vi "Configure Reference Wavelength.vi"(6 "Reference Wavelength (0 nm)":dbl, 7 "Channel (1: Channel 1)":i32(ring)=1 items=["All"=0, "Channel 1"=1, "Channel 1.1"=11, "Channel 1.2"=12, "Channel 1.3"=13, "Channel 1.4"=14, "Channel 2"=2, "Channel 2.1"=21, "Channel 2.2"=22, "Channel 2.3"=23, "Channel 2.4"=24, "Channel 3"=3, "Channel 3.1"=31, "Channel 3.2"=32, "Channel 3.3"=33, "Channel 3.4"=34, "Channel 4"=4, "Channel 4.1"=41, "Channel 4.2"=42, "Channel 4.3"=43, "Channel 4.4"=44], 8 "error in (no error)":errorcluster, 9 "Reference Action (0:Enable)":u16(ring) items=["Enable", "Disable", "Clear"], 10 "Sensor Number (1)":i32=1, 11 "VISA resource name":refnum<visa-resource-name>) -> (0 "error out":errorcluster, 3 "VISA resource name out":refnum<visa-resource-name>)   [LabVIEW 2015, in "Micron Optics sm130.lvlib"]
doc: "Configures the reference wavelength for a specified channel and sensor. Actions that could be performed on reference wavelength are enable/disable/clear."
uses:
  Micron Optics sm130.lvlib
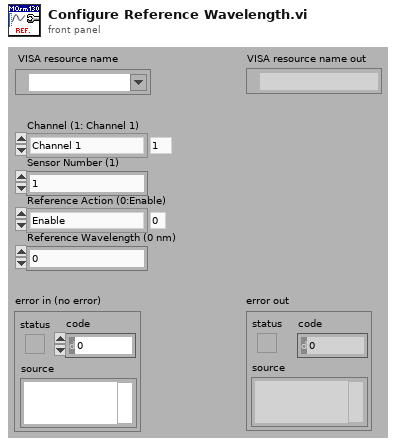
[diagram p1: front panel]
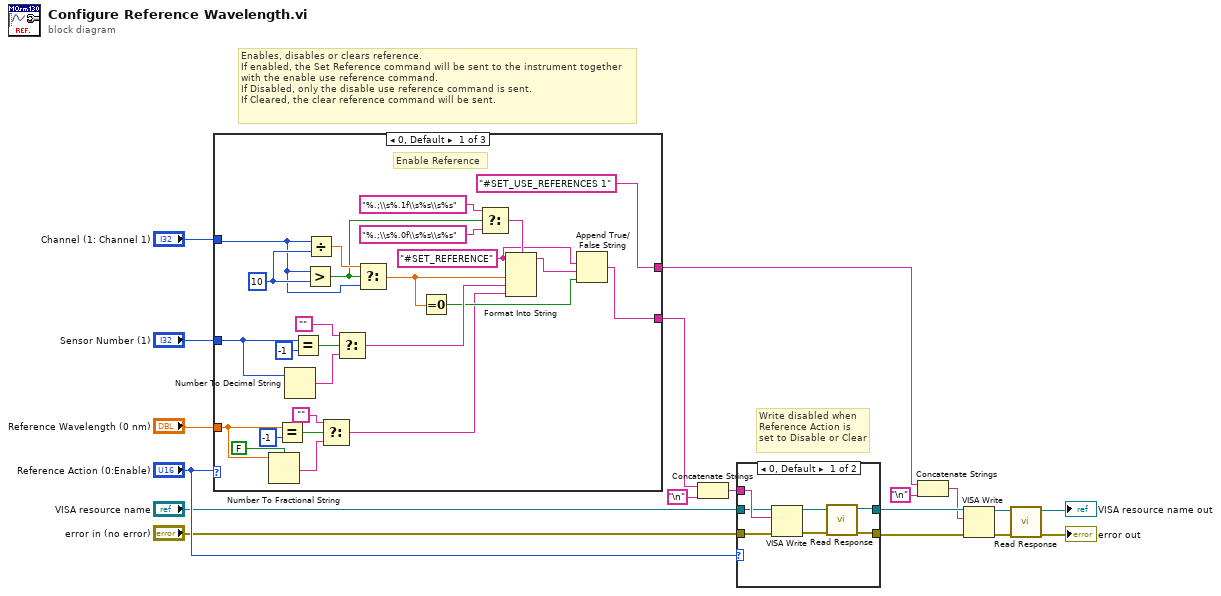
[diagram p0: block diagram]
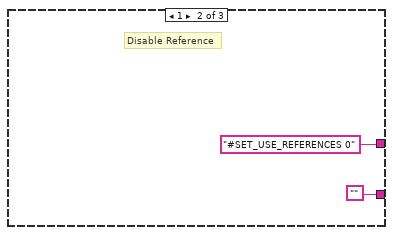
[diagram p3: hidden frame]
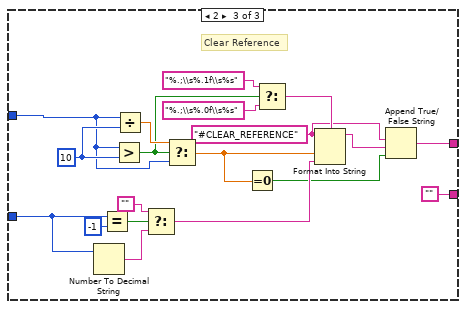
[diagram p4: hidden frame]
diagram:
  # "Enables, disables or clears reference. \nIf enabled, the Set Reference command will be sent to the instrument together with the enable use reference command. \nIf Disabled, only the disable use reference command is sent.\nIf Cleared, the clear reference command will be sent."
  # "Write disabled when Reference Action is set to Disable or Clear"
  n1 = case shown="0, Default" "Reference Action (0:Enable)" {
    tunnel: ["#SET_USE_REFERENCES 1" "#SET_USE_REFERENCES 0" w50] -> w1
    tunnel: "Channel (1: Channel 1)" -> [w29 _ w63]
    tunnel: "Sensor Number (1)" -> [w28 _ w49]
    tunnel: "Reference Wavelength (0 nm)" -> [w23 _ _]
    tunnel: [w21 "" ""] -> w5
    frame 0, Default {
      w32 = "#SET_REFERENCE" ("initial string")
      w42 = 10 ("y")
      # "Enable Reference"
      n2 = Number To Fractional String(use system decimal point (T)=FALSE, number=w23) -> (F-format string=w24:string)  [unwired: 2 in]
      n3 = Equal?(x=w23, y=-1) -> (x = y?=w26:bool)
      n4 = Number To Decimal String(number=w28) -> (decimal integer string=w30:string)  [unwired: 1 in]
      n5 = Equal?(x=w28, y=-1) -> (x = y?=w39:bool)
      n6 = Greater?(x=w29, y=w42) -> (0:w41:bool)
      n7 = Divide(x=w29, y=w42) -> (x/y=w43:dbl)
      n8 = Select(t="", s=w26, f=w24) -> (s? t:f=w22:string)
      n9 = Select(t="", s=w39, f=w30) -> (s? t:f=w38:string)
      n10 = Select(t=w43, s=w41, f=w29) -> (s? t:f=w34:dbl)
      n11 = Equal To 0?(x=w34) -> (x = 0?=w31:bool)
      n12 = Select(t="%.;\\s%.1f\\s%s\\s%s" ("format string"), s=w41, f="%.;\\s%.0f\\s%s\\s%s" ("format string")) -> (s? t:f=w35:string)
      n13 = Format Into String(format string=w35, initial string=w32, w34, w38, w22) -> (resulting string=w33:string)  [unwired: 1 in, 1 out]
      n14 = Append True/False String(1:w31, 2:w33, 3:w32) -> (0:w21:string)  [unwired: 1 in]
    }
    frame 1 {
      # "Disable Reference"
    }
    frame 2 {
      w52 = "#CLEAR_REFERENCE" ("initial string")
      w64 = 10 ("y")
      # "Clear Reference"
      n15 = Number To Decimal String(number=w49) -> (decimal integer string=w48:string)  [unwired: 1 in]
      n16 = Equal?(x=w49, y=-1) -> (x = y?=w60:bool)
      n17 = Greater?(x=w63, y=w64) -> (0:w62:bool)
      n18 = Divide(x=w63, y=w64) -> (x/y=w65:dbl)
      n19 = Select(t="", s=w60, f=w48) -> (s? t:f=w58:string)
      n20 = Select(t=w65, s=w62, f=w63) -> (s? t:f=w54:dbl)
      n21 = Equal To 0?(x=w54) -> (x = 0?=w51:bool)
      n22 = Select(t="%.;\\s%.1f\\s%s" ("format string"), s=w62, f="%.;\\s%.0f\\s%s" ("format string")) -> (s? t:f=w55:string)
      n23 = Format Into String(format string=w55, initial string=w52, w54, w58) -> (resulting string=w53:string)  [unwired: 1 in, 1 out]
      n24 = Append True/False String(1:w51, 2:w53, 3:w52) -> (0:w50:string)  [unwired: 1 in]
    }
  }
  n25 = Concatenate Strings(w5, "\n") -> (w6:string)
  n26 = case shown="0, Default" "Reference Action (0:Enable)" {
    tunnel: w6 -> [w72 _]
    tunnel: "VISA resource name" -> [w71 w74]
    tunnel: [w66 w74] -> w10
    tunnel: "error in (no error)" -> [w70 w73]
    tunnel: [w69 w73] -> w9
    frame 0, Default {
      n27 = VISA Write(VISA resource name=w71, write buffer=w72, error in (no error)=w70) -> (VISA resource name out=w68:refnum<visa-resource-name>, error out=w67:errorcluster)  [unwired: 1 out]
      n28 = call "Read Response.vi"("error in (no error)"=w67, "VISA resource name"=w68) -> ("error out"=w69:errorcluster, "VISA resource name out"=w66:refnum<visa-resource-name>)  [unwired: 7 in, 1 out]
    }
    frame 1, 2 {
    }
  }
  n29 = Concatenate Strings(w1, "\n") -> (w2:string)
  n30 = VISA Write(VISA resource name=w10, write buffer=w2, error in (no error)=w9) -> (VISA resource name out=w15:refnum<visa-resource-name>, error out=w14:errorcluster)  [unwired: 1 out]
  n31 = call "Read Response.vi"("error in (no error)"=w14, "VISA resource name"=w15) -> ("error out"=→"error out":errorcluster, "VISA resource name out"=→"VISA resource name out":refnum<visa-resource-name>)  [unwired: 7 in, 1 out]
